vi "InitCameraSeq.vi"(1 "Saving":bool, 5 "Scan.lvclass":refnum<class "Scan.lvclass">, 6 "error in":errorcluster, 7 "Progress":refnum<vi>, 8 "cropLines":dbl=1.0, 9 "DAQ in":refnum<class "DAQ.lvclass">) -> (0 "error out":errorcluster, 2 "Stop out":bool, 3 "Updated camera":T2, 4 "DAQ out":refnum<class "DAQ.lvclass">)   [LabVIEW 2017]
doc: "Creates, and edits acquisitions using the NI Vision Acquisition Express VI.\n\nThe NI Vision Acquisition Wizard is launched by placing the Express VI on the block diagram. Select an acquisition source and configure an acquisition using NI-IMAQ, NI-IMAQdx, or simulate an acquisition by reading an AVI or image files from a folder. After an acquisition is configured, select controls and indicators to be able to programmatically set in LabVIEW. Double-click the Vision Acquisition Express VI to edit the acquisition.\n\nNote: Any images created by the Express VI need to be disposed after use. Use the IMAQ Dispose.vi to cleanup the images output by the Express VI when they are no longer needed."
uses:
  classes/Scans/Scan.lvclass
  classes/HardwareObjects/DAQ/DAQ.lvclass
  <vilib>/vision/Image Controls.llb/IMAQ Image.ctl
  classes/Scans/Scan.lvclass/Scan.ctl
  classes/Scans/Read Total A-scans per frame.vi
  classes/Scans/Read Total B-Scans.vi
panel:
  out "IMAQ start time":dbl
  out "IMAQ start tic":dbl format="%_19f"
  out "IMAQ start toc":dbl format="%_19f"
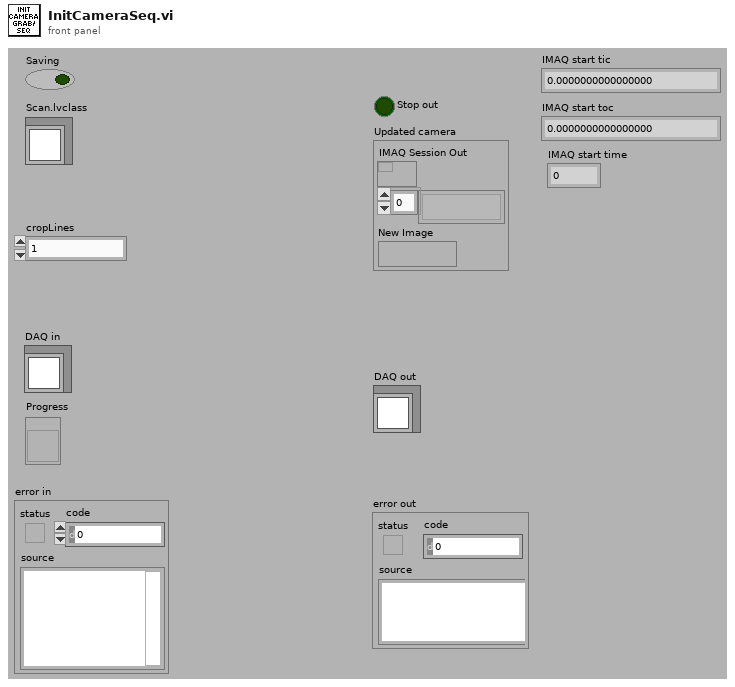
[diagram p1: front panel]
types:
  T1 = typedef "IMAQ Image.ctl" = refnum<image>
  T2 = cluster{"IMAQ Session Out":refnum<k11>, T1[], "New Image":T1}
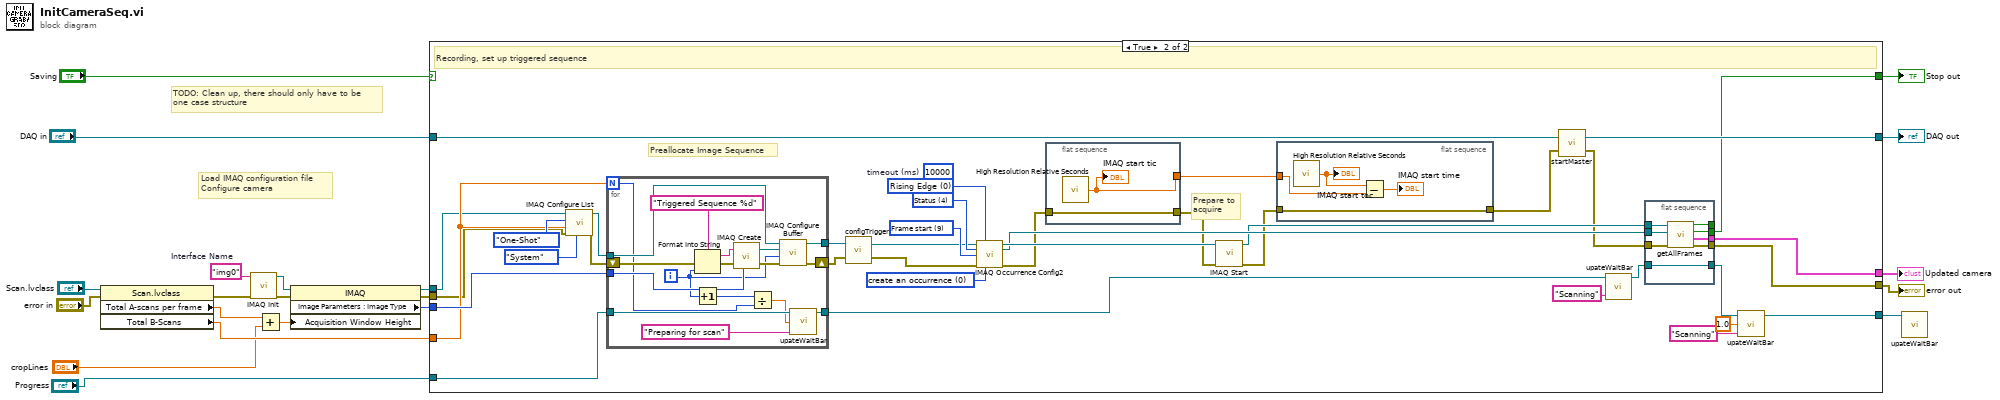
[diagram p0: block diagram]
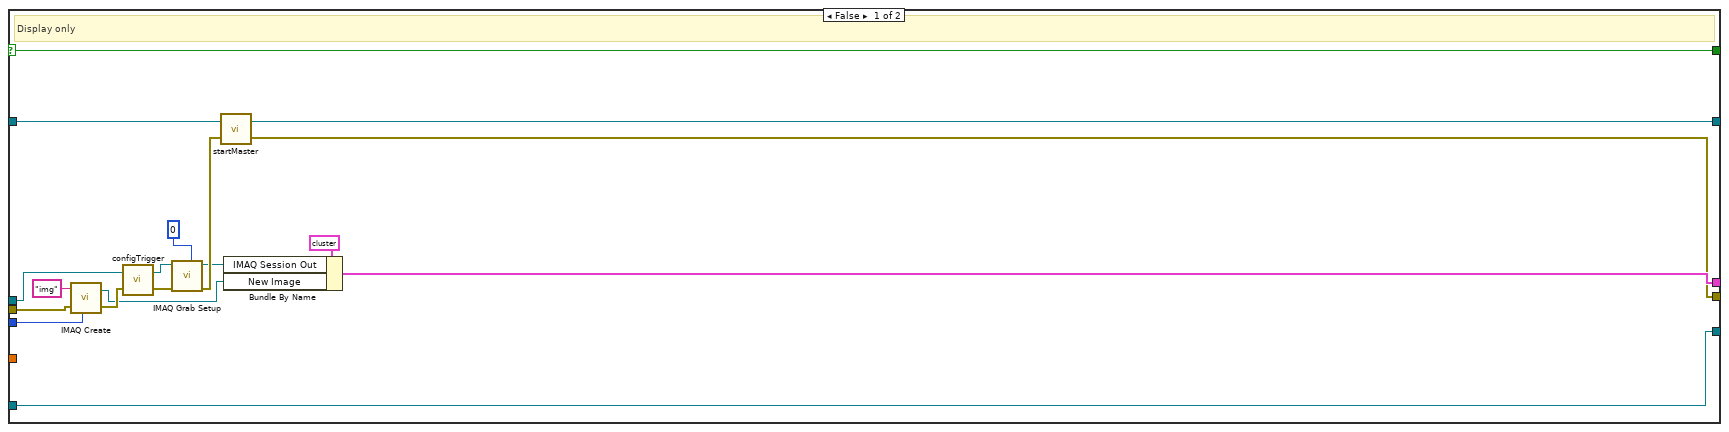
[diagram p2: hidden frame]
diagram:
  w18 = "img0"  # Interface Name
  # "TODO: Clean up, there should only have to be \none case structure"
  # "Load IMAQ configuration file\nConfigure camera"
  n1 = property class="Scan.lvclass"(reference="Scan.lvclass", error in="error in") -> (error out=w15:errorcluster, "Total A-scans per frame"=w2:dbl, "Total B-Scans"=w11:dbl)  [unwired: 1 out]
  n2 = call <vilib>:"IMAQ Init.vi"("error in (no error)"=w15, "Interface Name"=w18) -> ("error out"=w20:errorcluster, "IMAQ Session Out"=w14:refnum<k11>)  [unwired: 8 out]
  n3 = Add(x=w2, y="cropLines") -> (x+y=w3:dbl)
  n4 = property class="IMAQ"(reference=w14, error in=w20, "Acquisition Window Height"=w3) -> (reference out=w13:refnum<k11>, error out=w19:errorcluster, "Image Parameters : Image Type"=w21:u32)
  n5 = case shown="True" "Saving" {
    selector: "Saving" -> [w24 _]
    tunnel: w21 -> [w38 w75]
    tunnel: w19 -> [w39 w71]
    tunnel: w11 -> [_ w74]
    tunnel: w13 -> [w36 w73]
    tunnel: "Progress" -> [w22 w69]
    tunnel: "DAQ in" -> [w31 w60]
    tunnel: [w29 w59] -> w8
    tunnel: [w28 w54] -> w7
    tunnel: [w23 w53] -> w6
    tunnel: [w24 w52] -> w5
    tunnel: [w22 w45] -> w4
    frame False {
      # "Display only"
      n6 = call "IMAQ Create"("Image Name"="img", "Image Type"=w38, "error in (no error)"=w39) -> ("New Image"=w26:T1, "error out"=w35:errorcluster)  [unwired: 1 in, 1 out]
      n7 = call "configTrigger.vi"("error in (no error)"=w35, "IMAQ Session In"=w36) -> ("error out"=w33:errorcluster, "IMAQ Session Out"=w32:refnum<k11>)
      n8 = call <vilib>:"IMAQ Grab Setup.vi"("Channel"=0, "error in (no error)"=w33, "IMAQ Session In"=w32) -> ("error out"=w30:errorcluster, "IMAQ Session Out"=w25:refnum<k11>)  [unwired: 1 in, 6 out]
      n9 = call "startMaster.vi"("error in (no error)"=w30, "DAQ in"=w31) -> ("error out"=w23:errorcluster, "DAQ out"=w29:refnum<class "DAQ.lvclass">)
      n10 = Bundle By Name(cluster=T2 {"IMAQ Session Out"=refnum, [], "New Image"=refnum} ("Updated camera 2"), "IMAQ Session Out"=w25, "New Image"=w26) -> (w28:T2)
    }
    frame True {
      (unwired) 10000  # timeout (ms)
      w63 = u16 0 items=["create an occurrence", "clear all occurrences"] ("create/clear")
      w64 = u32 9 items=["Acquisition in progress"=15, "Acquisition done"=8, "Frame start"=9, "Frame done"=10, "Buffer Complete"=11] ("Status Signal")
      w65 = u32 4 items=["External", "RTSI ", "ISO In", "ISO Out", "Status"] ("Signal Type")
      w66 = u32 0 items=["Rising Edge", "Falling Edge"] ("Signal polarity")
      # "Prepare to\nacquire"
      # "Preallocate Image Sequence"
      # "Recording, set up triggered sequence"
      n11 = call <vilib>:"IMAQ Configure List.vi"("Memory Location"=enum16{"System", "Onboard"}."System", "error in (no error)"=w71, "Number of buffers"=w74, "Continuous?"=enum16{"One-Shot", "Continuous"}."One-Shot", "IMAQ Session In"=w73) -> ("error out"=w70:errorcluster, "IMAQ Session Out"=w72:refnum<k11>)  [unwired: 1 in, 4 out]
      n12 = for {
        N: w74 -> [w94]
        tunnel: [w108] -> w68
        tunnel: w72 -> [w104]
        tunnel: w75 -> [w106]
        shift-right: [w107] -> w67
        shift-left: w70 -> [w100]
        tunnel: w69 -> [w98]
        tunnel: [w92] -> w51
        i -> [w96]
        n13 = Format Into String(format string="Triggered Sequence %d", error in=w100, w96) -> (resulting string=w101:string, error out=w99:errorcluster)  [unwired: 1 in]
        n14 = Increment(x=w96) -> (x+1=w95:i32)
        n15 = call "IMAQ Create"("Image Name"=w101, "Image Type"=w106, "error in (no error)"=w99) -> ("New Image"=w103:T1, "error out"=w105:errorcluster)  [unwired: 1 in, 1 out]
        n16 = Divide(x=w95, y=w94) -> (x/y=w93:dbl)
        n17 = call <vilib>:"IMAQ Configure Buffer.vi"("error in (no error)"=w105, "Buffer Number"=w96, "Image In"=w103, "IMAQ Session In"=w104) -> ("error out"=w107:errorcluster, "IMAQ Session Out"=w108:refnum<k11>)  [unwired: 2 in, 4 out]
        n18 = call "upateWaitBar.vi"("waitbar text"="Preparing for scan", "waitbar value [0,1]"=w93, "Progress"=w98) -> ("Updated Progress"=w92:refnum<vi>)  [unwired: 2 in]
      }
      n19 = call "configTrigger.vi"("error in (no error)"=w67, "IMAQ Session In"=w68) -> ("error out"=w61:errorcluster, "IMAQ Session Out"=w62:refnum<k11>)
      n20 = call <vilib>:"IMAQ Occurrence Config2.vi"("IMAQ Session In"=w62, "Signal polarity"=w66, "Signal Type"=w65, "Status Signal"=w64, "error in (no error)"=w61, "create/clear"=w63) -> ("IMAQ Session Out"=w58:refnum<k11>, "occurrence"=w57:refnum<k4>, "error out"=w44:errorcluster)  [unwired: 7 in]
      n21 = flat-sequence {
        tunnel: w44 -> [w83]
        tunnel: [w83] -> w43
        tunnel: [w82] -> w40
        frame #0 {
          n22 = call <vilib>:"High Resolution Relative Seconds.vi"() -> ("relative seconds"=w82:dbl)
          "IMAQ start tic" <- w82
        }
      }
      n23 = call <vilib>:"IMAQ Start.vi"("error in (no error)"=w43, "IMAQ Session In"=w58) -> ("error out"=w42:errorcluster, "IMAQ Session Out"=w56:refnum<k11>)  [unwired: 8 out]
      n24 = flat-sequence {
        tunnel: w42 -> [w81]
        tunnel: [w81] -> w41
        tunnel: w40 -> [w79]
        frame #0 {
          n25 = call <vilib>:"High Resolution Relative Seconds.vi"() -> ("relative seconds"=w80:dbl)
          "IMAQ start toc" <- w80
          n26 = Subtract(x=w80, y=w79) -> (x-y=→"IMAQ start time":dbl)
        }
      }
      n27 = call "startMaster.vi"("error in (no error)"=w41, "DAQ in"=w60) -> ("error out"=w55:errorcluster, "DAQ out"=w59:refnum<class "DAQ.lvclass">)
      n28 = call "upateWaitBar.vi"("waitbar text"="Scanning", "Progress"=w51) -> ("Updated Progress"=w50:refnum<vi>)  [unwired: 3 in]
      n29 = flat-sequence {
        tunnel: w57 -> [w91]
        tunnel: w56 -> [w90]
        tunnel: w55 -> [w89]
        tunnel: [w88] -> _
        tunnel: [w87] -> w54
        tunnel: [w86] -> w53
        tunnel: [w85] -> w52
        tunnel: w50 -> [w84]
        tunnel: [w84] -> w48
        frame #0 {
          n30 = call "getAllFrames.vi"("error in (no error)"=w89, "1st occurrence"=w91, "IMAQ Session In"=w90) -> ("error out"=w86:errorcluster, "Updated camera"=w87:T2, "Finished Acquisition"=w85:bool, "Encountered Trigger"=w88:bool)  [unwired: 5 in]
        }
      }
      n31 = call "upateWaitBar.vi"("waitbar text"="Scanning", "waitbar value [0,1]"=sgl 1.0, "Progress"=w48) -> ("Updated Progress"=w45:refnum<vi>)  [unwired: 2 in]
    }
  }
  "DAQ out" <- w8
  "Updated camera" <- w7
  "error out" <- w6
  "Stop out" <- w5
  n32 = call "upateWaitBar.vi"("Progress"=w4) -> ()  [unwired: 4 in, 1 out]
